vi "Set current stack.vi"(8 "error in (no error)":errorcluster, 10 "Current stack":u16, 11 "Tomo in":refnum<class "Tomo.lvclass">) -> (0 "error out":errorcluster, 3 "Tomo out":refnum<class "Tomo.lvclass">)   [LabVIEW 2012, in "Tomo.lvclass"]
uses:
  Tomo.lvclass
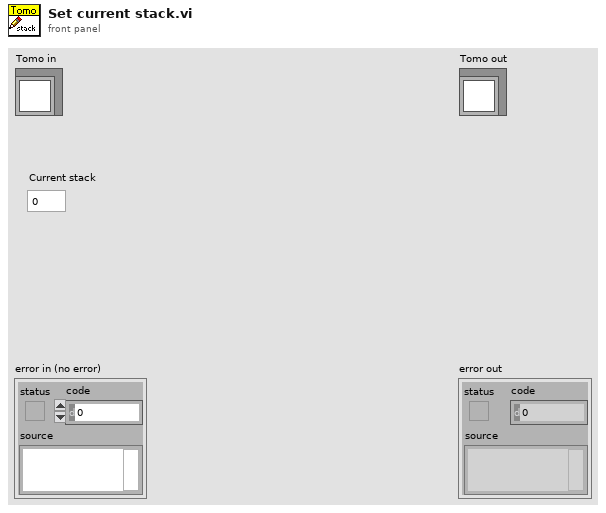
[diagram p1: front panel]
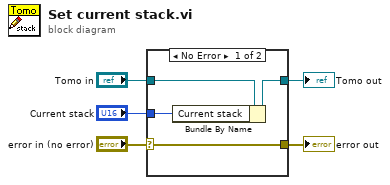
[diagram p0: block diagram]
diagram:
  n1 = case shown="No Error" "error in (no error)" {
    selector: "error in (no error)" -> [w9 w11]
    tunnel: [w9 w11] -> w4
    tunnel: [w7 w10] -> w2
    tunnel: "Tomo in" -> [w8 w10]
    tunnel: "Current stack" -> [w6 _]
    frame No Error {
      n2 = Bundle By Name(cluster=w8, "Current stack"=w6) -> (w7:refnum<class "Tomo.lvclass">)
    }
    frame Error {
    }
  }
  "error out" <- w4
  "Tomo out" <- w2
